vi "UI_ShowIn_FreeWindow.vi"(8 "error in (no error)":errorcluster, 9 "Panel Bounds (if Std)":T1, 10 "Standard/Max (T=Max)":bool, 11 "UI_Actor in":refnum<class "UI_Actor.lvclass">) -> (0 "error out":errorcluster, 3 "UI_Actor out":refnum<class "UI_Actor.lvclass">)   [LabVIEW 2020, in "UI_Actor.lvlib" / "UI_Actor.lvclass"]
uses:
  UI_Actor.lvclass
  <vilib>/Utility/miscctls.llb/LVRectTypeDef.ctl
  UI_Actor.lvclass/UI_Actor.ctl
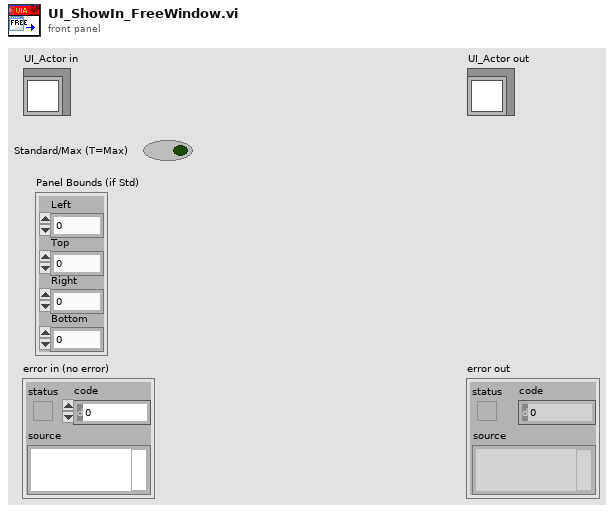
[diagram p1: front panel]
types:
  T1 = typedef "LVRectTypeDef.ctl" = cluster{"Left":i16, "Top":i16, "Right":i16, "Bottom":i16}
  T2 = enum32{"Invalid", "Standard", "Closed", "Hidden", "Minimized", "Maximized"}
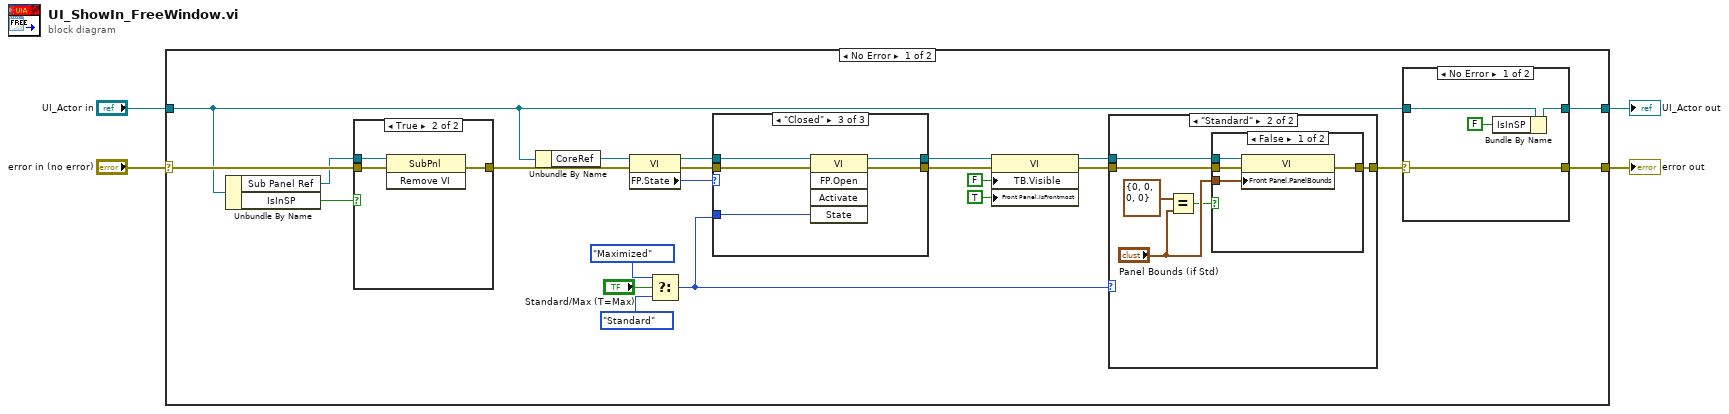
[diagram p0: block diagram]
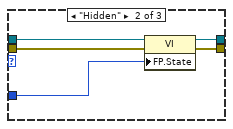
[diagram p7: hidden frame]
diagram:
  n1 = case shown="No Error" "error in (no error)" {
    selector: "error in (no error)" -> [w17 w62]
    tunnel: [w14 w62] -> w3
    tunnel: [w12 w61] -> w1
    tunnel: "UI_Actor in" -> [w13 w61]
    frame No Error {
      n2 = Unbundle By Name(w13) -> ("Sub Panel Ref"=w16:refnum<vi>, "IsInSP"=w18:bool)
      n3 = case shown="True" w18 {
        tunnel: w17 -> [w45 w48]
        tunnel: w16 -> [_ w47]
        tunnel: [w45 w46] -> w15
        frame False {
        }
        frame True {
          n4 = invoke on="Invoke Node" class="SubPnl" method="Remove VI"(reference=w47, error in=w48) -> (error out=w46:errorcluster)  [unwired: 1 in, 2 out]
        }
      }
      n5 = Unbundle By Name(w13) -> ("CoreRef"=w20:refnum<vi>)
      n6 = property class="VI"(reference=w20, error in=w15) -> (reference out=w25:refnum<vi>, error out=w22:errorcluster, "FP.State"=w26:T2)
      n7 = Select(t=T2."Maximized" ("State (maximized)"), s="Standard/Max (T=Max)", f=T2."Standard" ("State (maximized)")) -> (s? t:f=w6:T2)
      n8 = case shown="\"Closed\"" w26 {
        tunnel: [w50 w54 w59] -> w24
        tunnel: w25 -> [w50 w55 w60]
        tunnel: w22 -> [w49 w53 w57]
        tunnel: [w49 w52 w58] -> w21
        tunnel: w6 -> [_ w51 w56]
        frame Default {
        }
        frame "Hidden" {
          n9 = property class="VI"(reference=w55, error in=w53, "FP.State"=w51) -> (reference out=w54:refnum<vi>, error out=w52:errorcluster)
        }
        frame "Closed" {
          n10 = invoke class="VI" method="FP.Open"(reference=w60, error in=w57, "State"=w56) -> (reference out=w59:refnum<vi>, error out=w58:errorcluster)  [unwired: 2 in, 3 out]
        }
      }
      n11 = property class="VI"(reference=w24, error in=w21, "TB.Visible"=FALSE ("Tool Bar:Visible"), "Front Panel.IsFrontmost"=TRUE ("Front Panel Window:Is Frontmost")) -> (reference out=w9:refnum<vi>, error out=w10:errorcluster)
      n12 = case shown="\"Standard\"" w6 {
        tunnel: [w27 w31] -> w11
        tunnel: w10 -> [w27 w33]
        tunnel: w9 -> [_ w32]
        frame Default {
        }
        frame "Standard" {
          n13 = Equal?(x=T1 {"Left"=0, "Top"=0, "Right"=0, "Bottom"=0}, y="Panel Bounds (if Std)") -> (x = y?=w28:bool)
          n14 = case shown="False" w28 {
            tunnel: w33 -> [w37 w38]
            tunnel: w32 -> [w36 _]
            tunnel: [w35 w38] -> w31
            tunnel: "Panel Bounds (if Std)" -> [w34 _]
            frame False {
              n15 = property class="VI"(reference=w36, error in=w37, "Front Panel.PanelBounds"=w34) -> (error out=w35:errorcluster)  [unwired: 1 out]
            }
            frame True {
            }
          }
        }
      }
      n16 = case shown="No Error" w11 {
        selector: w11 -> [w41 w44]
        tunnel: [w41 w44] -> w14
        tunnel: w13 -> [w42 w43]
        tunnel: [w40 w43] -> w12
        frame No Error {
          n17 = Bundle By Name(cluster=w42, "IsInSP"=FALSE ("Window management.IsInSP")) -> (w40:refnum<class "UI_Actor.lvclass">)
        }
        frame Error {
        }
      }
    }
    frame Error {
    }
  }
  "error out" <- w3
  "UI_Actor out" <- w1
